vi "Logging Message Loop.vi"(8 "error in (no error)":errorcluster, 10 "Data Queue":refnum<queue>, 11 "Message Queues":T1) -> (0 "error out":errorcluster)   [LabVIEW 2017, in "Logging.lvlib"]
doc: "The message loop subVI to handle messages pertaining to logging data."
uses:
  Logging.lvlib
  support/Message Queue/All Message Queues.ctl
  support/Message Queue/Message Cluster.ctl
  Logging Configuration.ctl
  support/Message Queue/Enqueue Message (Single).vi
  <vilib>/Utility/error.llb/Error Cluster From Error Code.vi
  <vilib>/ErrorRing/Error Ring.xnode
  support/Message Queue/Message Queue.lvlib
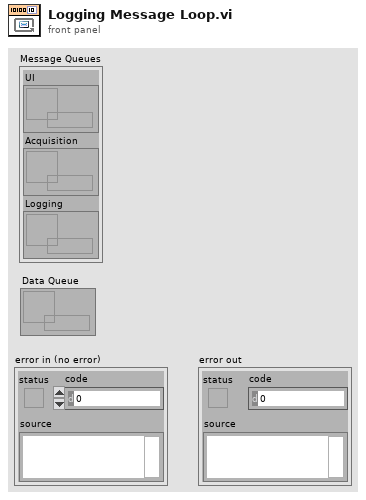
[diagram p1: front panel]
types:
  T1 = typedef "Message Queue.lvlib/All Message Queues.ctl" = cluster{"UI":refnum<queue>, "Acquisition":refnum<queue>, "Logging":refnum<queue>}
  T2 = typedef "Logging.lvlib/Logging Configuration.ctl" = cluster{"Log File Base Path":path, "TDMS File Reference":refnum<k34>, "Channel names":string[], "Author":string, "Description":string}
  T3 = enum16{"open", "open or create", "create or replace", "create", "open (read-only)"}
  T4 = cluster{"single precision float":waveform(sgl)[]}[]
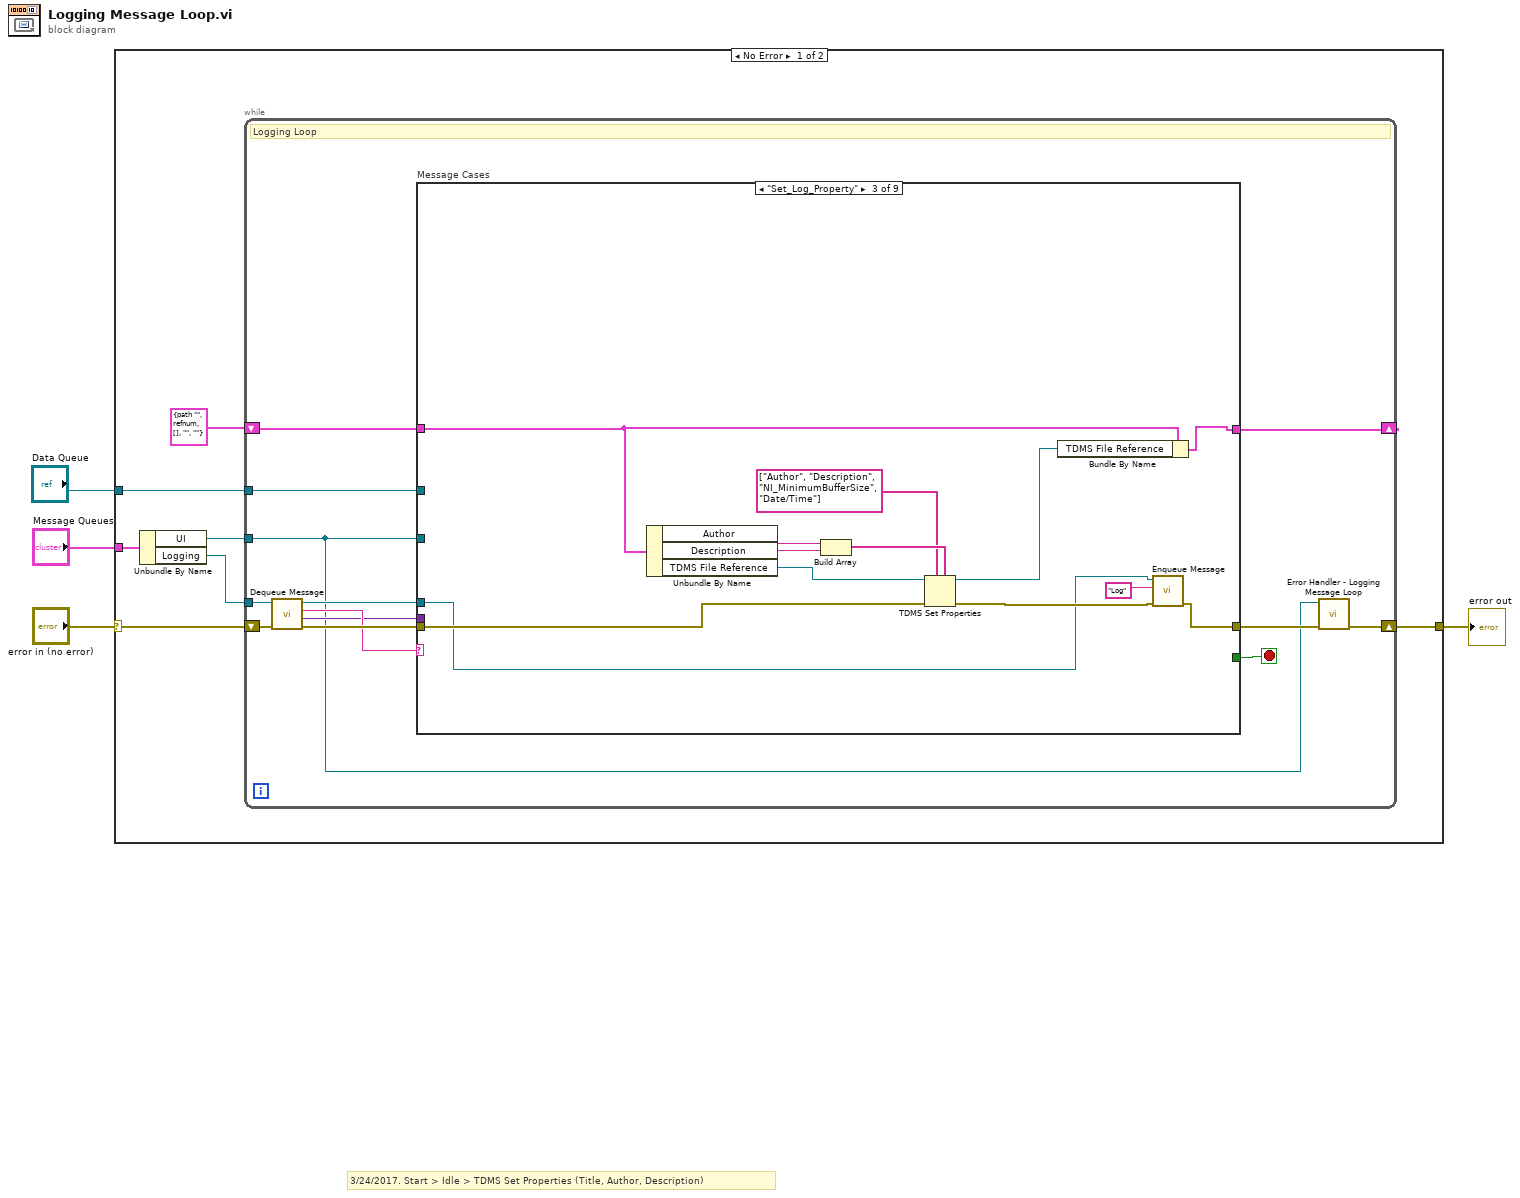
[diagram p0: block diagram]
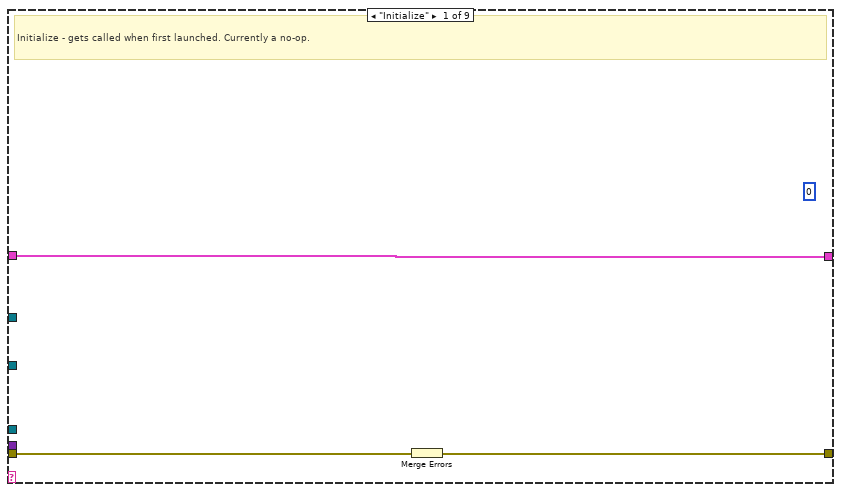
[diagram p2: hidden frame]
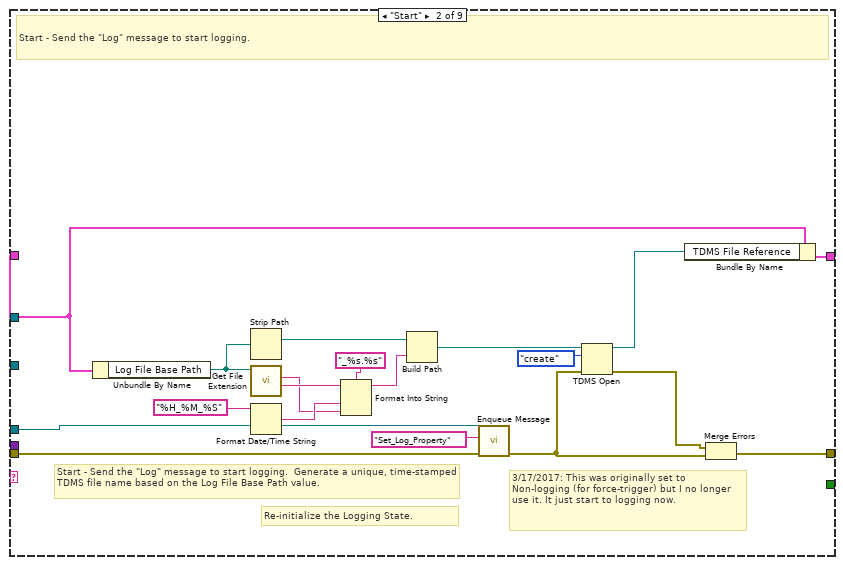
[diagram p3: hidden frame]
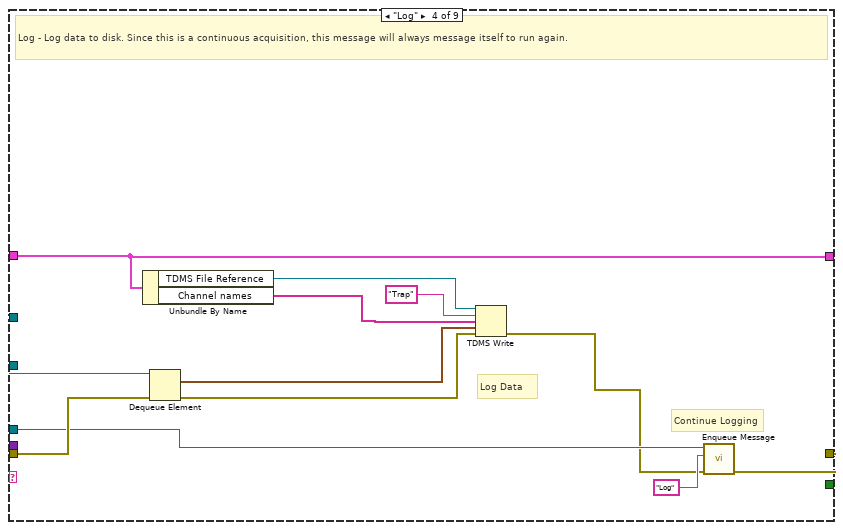
[diagram p4: hidden frame]
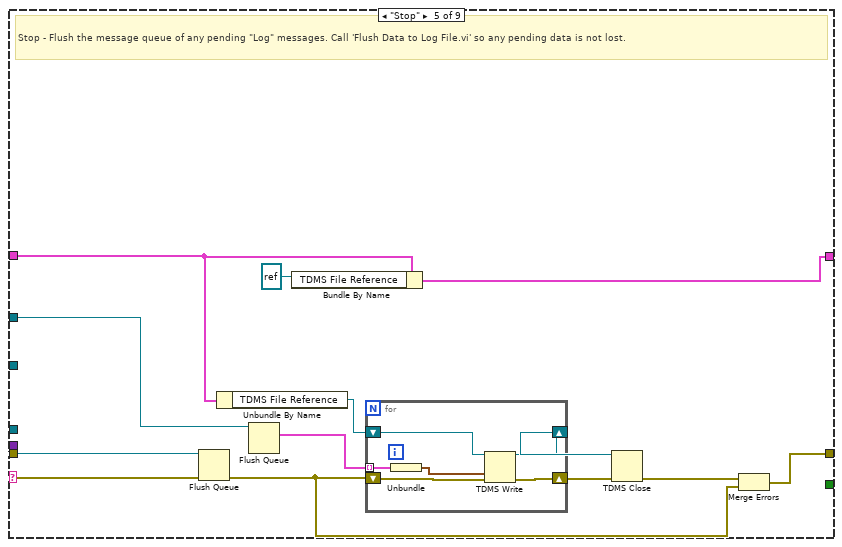
[diagram p5: hidden frame]
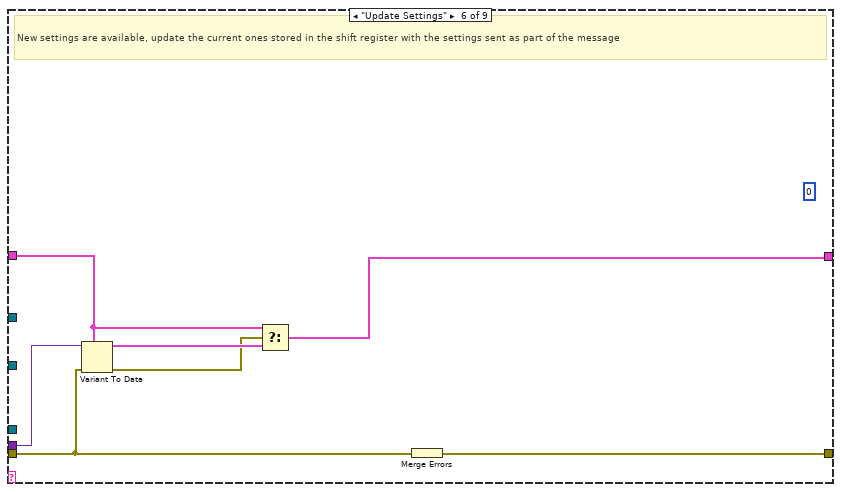
[diagram p6: hidden frame]
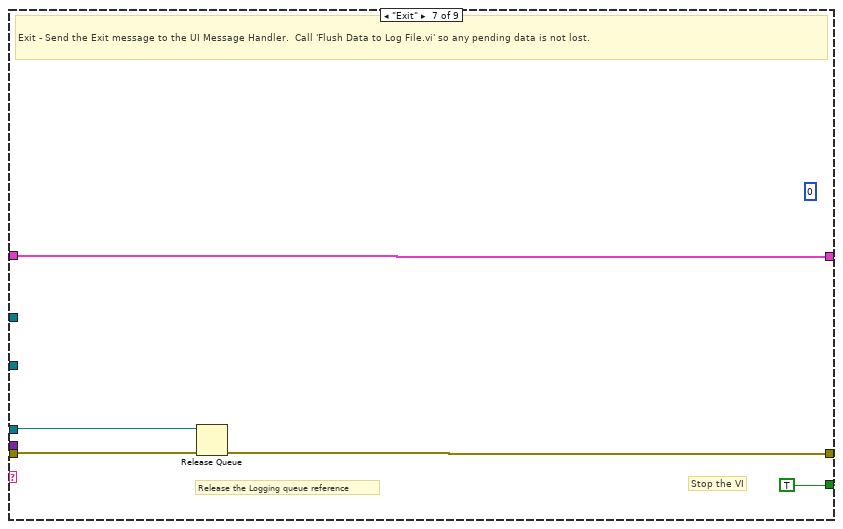
[diagram p7: hidden frame]
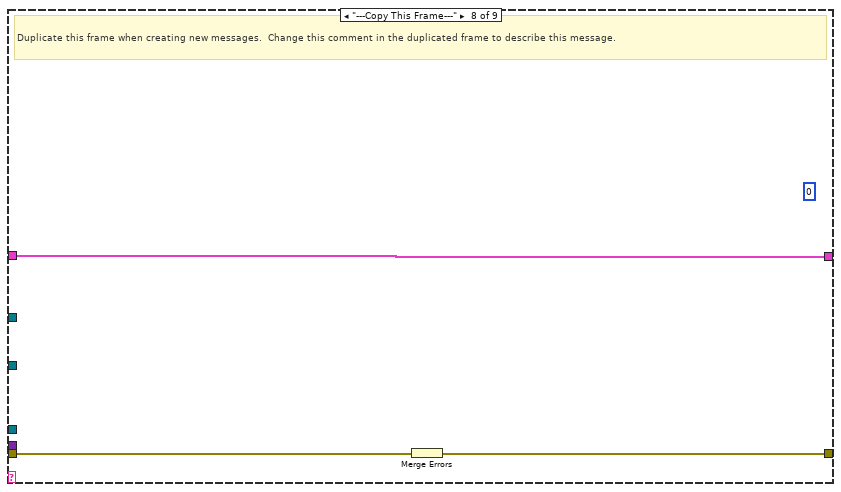
[diagram p8: hidden frame]
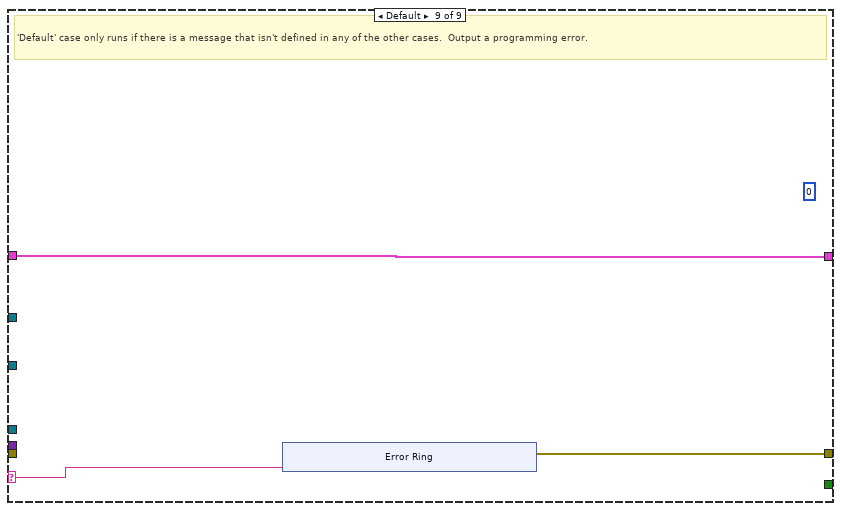
[diagram p9: hidden frame]
diagram:
  # "3/24/2017. Start > Idle > TDMS Set Properties (Title, Author, Description)"
  n1 = case shown="No Error" "error in (no error)" {
    selector: "error in (no error)" -> [w7 w116]
    tunnel: "Message Queues" -> [w11 _]
    tunnel: [w9 w116] -> w3
    tunnel: "Data Queue" -> [w6 _]
    frame No Error {
      n2 = Unbundle By Name(w11) -> ("UI"=w5:refnum<queue>, "Logging"=w10:refnum<queue>)
      n3 = while {
        tunnel: w10 -> [w16]
        shift-right: [w23] -> _
        shift-left: T2 {"Log File Base Path"=path "", "TDMS File Reference"=refnum, "Channel names"=[], "Author"="", "Description"=""} ("Logging Configuration") -> [w24]
        shift-right: [w13] -> w9
        shift-left: w7 -> [w21]
        tunnel: w5 -> [w12]
        tunnel: w6 -> [w15]
        stop <- w22 stop-if-true
        # "Logging Loop"
        n4 = call "Dequeue Message.vi"("error in (no error)"=w21, "Message Queue"=w16) -> ("error out"=w20:errorcluster, "Message Data"=w18:variant, "Message"=w19:string, "dup Message Queue"=w17:refnum<queue>)  [unwired: 6 in]
        n5 = case "Message Cases" shown="\"Set_Log_Property\"" w19 {
          selector: w19 -> [_ _ _ _ _ _ _ _ w106]
          tunnel: w17 -> [_ w45 w48 w67 w82 _ w100 _ _]
          tunnel: w20 -> [w25 w44 w51 w69 w83 w91 w101 w105 _]
          tunnel: [w27 w46 w49 w71 w84 w97 w98 w103 w107] -> w14
          tunnel: w24 -> [w26 w43 w53 w63 w79 w95 w99 w104 w108]
          tunnel: [w26 w42 w52 w63 w81 w92 w99 w104 w108] -> w23
          tunnel: [_ _ _ _ _ _ TRUE _ _] -> w22
          tunnel: w18 -> [_ _ _ _ _ w96 _ _ _]
          tunnel: w12 -> [_ _ _ _ _ _ _ _ _]
          tunnel: w15 -> [_ _ _ w68 w78 _ _ _ _]
          frame "Initialize" {
            (unwired) u32 0
            # "Initialize - gets called when first launched. Currently a no-op."
            n6 = Merge Errors(w25) -> (w27:errorcluster)
          }
          frame "Start" {
            # "3/17/2017: This was originally set to Non-logging (for force-trigger) but I no longer use it. It just start to logging now."
            # "Re-initialize the Logging State."
            # "Start - Send the \"Log\" message to start logging.  Generate a unique, time-stamped TDMS file name based on the Log File Base Path value."
            # "Start - Send the \"Log\" message to start logging."
            n7 = Unbundle By Name(w43) -> ("Log File Base Path"=w39:path)
            n8 = Strip Path(path=w39) -> (stripped path=w38:path)  [unwired: 1 out]
            n9 = call <vilib>:"Get File Extension.vi"("file"=w39) -> ("filename without extension"=w37:string, "lowercase file extension"=w34:string)  [unwired: 6 in, 3 out]
            n10 = Format Date/Time String(time format string (%c)="%H_%M_%S") -> (date/time string=w35:string)  [unwired: 2 in]
            n11 = Format Into String(format string="_%s.%s", initial string=w37, w35, w34) -> (resulting string=w33:string)  [unwired: 1 in, 1 out]
            n12 = Build Path(base path=w38, name or relative path=w33) -> (appended path=w30:path)
            n13 = call-poly "Enqueue Message.vi"("error in (no error)"=w44, "Message"="Set_Log_Property", "Message Queue"=w45) -> ("error out"=w31:errorcluster)  [unwired: 7 in, 1 out]
            n14 = TDMS Open(8:w31, 10:T3."create" ("operation (0:open)"), 11:w30) -> (0:w28:errorcluster, 3:w29:refnum<k34>)  [unwired: 4 in]
            n15 = Bundle By Name(cluster=w43, "TDMS File Reference"=w29) -> (w42:T2)
            n16 = Merge Errors(w28, w31) -> (w46:errorcluster)
          }
          frame "Set_Log_Property" {
            n17 = Unbundle By Name(w53) -> ("Author"=w57:string, "Description"=w56:string, "TDMS File Reference"=w58:refnum<k34>)
            n18 = Build Array(w57, w56) -> (w55:string[])
            n19 = TDMS Set Properties(5:w55, 7:string[] ["Author", "Description", "NI_MinimumBufferSize", "Date/Time"] ("property names"), 8:w51, 11:w58) -> (0:w50:errorcluster, 3:w54:refnum<k34>)  [unwired: 2 in, 2 out]
            n20 = Bundle By Name(cluster=w53, "TDMS File Reference"=w54) -> (w52:T2)
            n21 = call-poly "Enqueue Message.vi"("error in (no error)"=w50, "Message"="Log", "Message Queue"=w48) -> ("error out"=w49:errorcluster)  [unwired: 7 in, 1 out]
          }
          frame "Log" {
            # "Continue Logging"
            # "Log Data"
            # "Log - Log data to disk. Since this is a continuous acquisition, this message will always message itself to run again."
            n22 = Unbundle By Name(w63) -> ("TDMS File Reference"=w66:refnum<k34>, "Channel names"=w60:string[])
            n23 = Dequeue Element(queue=w68, error in (no error)=w69) -> (element=w64:waveform(sgl)[], error out=w65:errorcluster)  [unwired: 1 in, 2 out]
            n24 = TDMS Write(0:w66, 5:"Trap" ("group name in (Untitled)"), 7:w60, 9:w64, 11:w65) -> (15:w62:errorcluster)  [unwired: 1 in, 3 out]
            n25 = call-poly "Enqueue Message.vi"("error in (no error)"=w62, "Message"="Log", "Message Queue"=w67) -> ("error out"=w71:errorcluster)  [unwired: 7 in, 1 out]
          }
          frame "Stop" {
            # "Stop - Flush the message queue of any pending \"Log\" messages. Call 'Flush Data to Log File.vi' so any pending data is not lost."
            n26 = Flush Queue(queue=w82, error in (no error)=w83) -> (error out=w73:errorcluster)  [unwired: 2 out]
            n27 = Unbundle By Name(w79) -> ("TDMS File Reference"=w75:refnum<k34>)
            n28 = Flush Queue(queue=w78) -> (remaining elements=w77:T4)  [unwired: 1 in, 2 out]
            n29 = Bundle By Name(cluster=w79, "TDMS File Reference"=refnum<k34> refnum ("tdms file out")) -> (w81:T2)
            n30 = for {
              shift-right: [w87] -> w74
              shift-left: w75 -> [w88]
              shift-right: [w89] -> w76
              shift-left: w73 -> [w90]
              tunnel: w77 -> [w86] mode=indexing
              n31 = Unbundle(w86) -> ("single precision float"=w85:waveform(sgl)[])
              n32 = TDMS Write(0:w88, 9:w85, 11:w90) -> (4:w87:refnum<k34>, 15:w89:errorcluster)  [unwired: 3 in, 2 out]
            }
            n33 = TDMS Close(8:w76, 11:w74) -> (0:w72:errorcluster)  [unwired: 1 out]
            n34 = Merge Errors(w72, w73) -> (w84:errorcluster)
          }
          frame "Update Settings" {
            (unwired) u32 0
            # "New settings are available, update the current ones stored in the shift register with the settings sent as part of the message"
            n35 = Variant To Data(error in=w91, type=w95, Variant=w96) -> (data=w94:T2, error out=w93:errorcluster)
            n36 = Select(t=w95, s=w93, f=w94) -> (s? t:f=w92:T2)
            n37 = Merge Errors(w91) -> (w97:errorcluster)
          }
          frame "Exit" {
            (unwired) u32 0
            # "Release the Logging queue reference"
            # "Stop the VI"
            # "Exit - Send the Exit message to the UI Message Handler.  Call 'Flush Data to Log File.vi' so any pending data is not lost."
            n38 = Release Queue(queue=w100, error in (no error)=w101) -> (error out=w98:errorcluster)  [unwired: 1 in, 2 out]
          }
          frame "---Copy This Frame---" {
            (unwired) u32 0
            # "Duplicate this frame when creating new messages.  Change this comment in the duplicated frame to describe this message."
            n39 = Merge Errors(w105) -> (w103:errorcluster)
          }
          frame Default {
            (unwired) u32 0
            # "'Default' case only runs if there is a message that isn't defined in any of the other cases.  Output a programming error."
            n40 = xnode "Error Ring"("parameter 0"=w106) -> ("error out"=w107:errorcluster)
          }
        }
        n41 = call "Error Handler - Logging Message Loop.vi"("error in (no error)"=w14, "Message Queue"=w12) -> ("dup error in"=w13:errorcluster)  [unwired: 8 in, 1 out]
      }
    }
    frame Error {
    }
  }
  "error out" <- w3
